vi "Initialize.vi"(8 "error in (no error)":errorcluster, 9 "VISA Com Port":refnum<visa-resource-name>, 10 "Serial Device Brand":T1, 11 "Simulado in":refnum<class "Simulado.lvclass">) -> (0 "error out":errorcluster, 3 "Simulado out":refnum<class "Simulado.lvclass">)   [LabVIEW 2020, in "Simulado.lvclass"]
doc: "Método heredado del padre con un override"
uses:
  Simulado.lvclass
  Controles/Brand combobox.ctl
  Abstract/Serial device/Serial device.lvclass
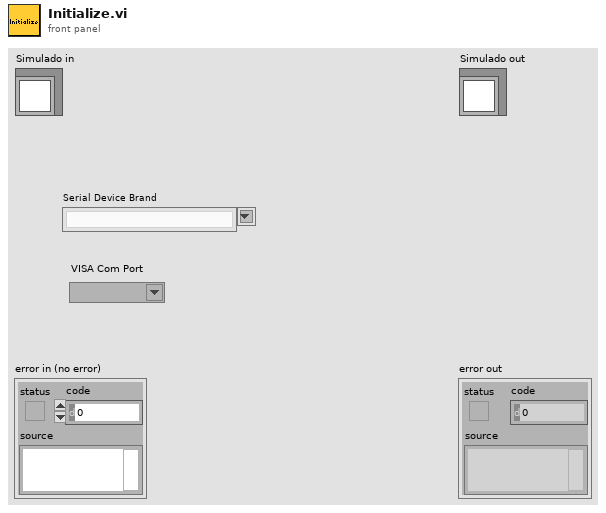
[diagram p1: front panel]
types:
  T1 = typedef "Serial device.lvclass/Brand combobox.ctl" = string
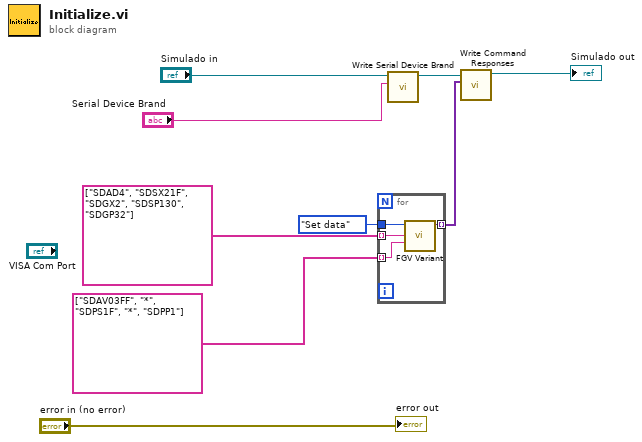
[diagram p0: block diagram]
diagram:
  n1 = for {
    tunnel: enum16{"Reset data", "Set data", "Get data"}."Set data" ("Functions") -> [w13]
    tunnel: string[] ["SDAD4", "SDSX21F", "SDGX2", "SDSP130", "SDGP32"] ("Response to save") -> [w12] mode=indexing
    tunnel: string[] ["SDAV03FF", "*", "SDPS1F", "*", "SDPP1"] ("Response to save") -> [w11] mode=indexing
    tunnel: [w10] -> w2 mode=indexing
    n2 = call "FGV Variant.vi"("Response to save"=w11, "Command"=w12, "Functions"=w13) -> ("Variant"=w10:variant)  [unwired: 7 in, 1 out]
  }
  n3 = call-dynamic "Write Serial Device Brand.vi"("Serial Device Brand"="Serial Device Brand", "Serial device in"="Simulado in") -> ("Serial device out"=w5:refnum<class "Simulado.lvclass">)  [unwired: 8 in, 1 out]
  n4 = call-dynamic "Write Command Responses.vi"("Command Responses"=w2, "Simulado in"=w5) -> ("Simulado out"=→"Simulado out":refnum<class "Simulado.lvclass">)  [unwired: 8 in, 1 out]
  "error out" <- "error in (no error)"
